vi "MassCompile7.1.vi"(1 "Directory To Compile":path) -> (0 "error out":errorcluster)   [LabVIEW 2014]
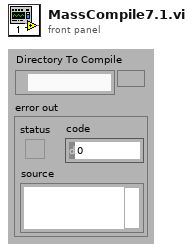
[diagram p1: front panel]
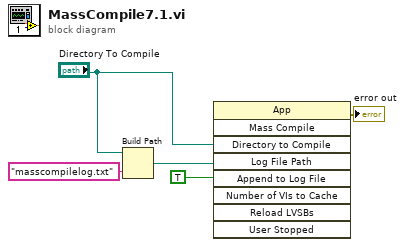
[diagram p0: block diagram]
diagram:
  n1 = Build Path(base path="Directory To Compile", name or relative path="masscompilelog.txt") -> (appended path=w5:path)
  n2 = invoke class="App" method="Mass Compile"("Directory to Compile"="Directory To Compile", "Log File Path"=w5, "Append to Log File"=TRUE) -> (error out=→"error out":errorcluster)  [unwired: 6 in, 8 out]
